vi "channel cluster to array.vi"(11 "input cluster":T1 {"Vfile (V)" format="%.1f V"; "Vswmax (V)" format="%#_g V"; "Iset (A)" format="%.2pA"; "Imon (A)" format="%.2pA"; "Vset (V)" format="%#_g V"; "Vmon (V)" format="%.1f V"}) -> (3 "Array":string[](array[string]))   [LabVIEW 2018]
uses:
  channel_cluster.ctl
  bool to string small.vi
  dbl to fr string small.vi
  i32 to dec string small.vi
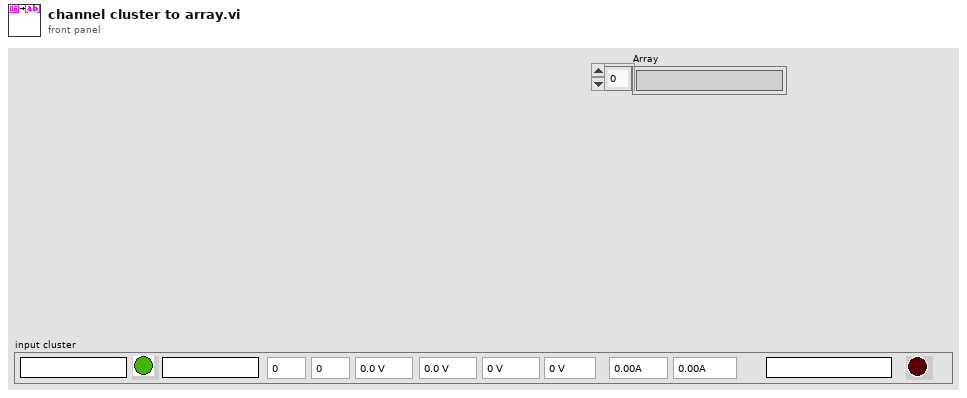
[diagram p1: front panel]
types:
  T1 = typedef "channel_cluster.ctl" = cluster{"Channel Name":string, "Crate":i32, "Card Type":string, "Card":i32, "Channel":i32, "Status Icon":picture, "Vmon (V)":dbl, "Vset (V)":dbl, "Imon (A)":dbl, "Iset (A)":dbl, "Timestamp":string, "ON/OFF":bool, "Status":string, "Vswmax (V)":dbl, "Flag":bool, "Vfile (V)":dbl, "Error Logged":bool[], "enable_file":bool}
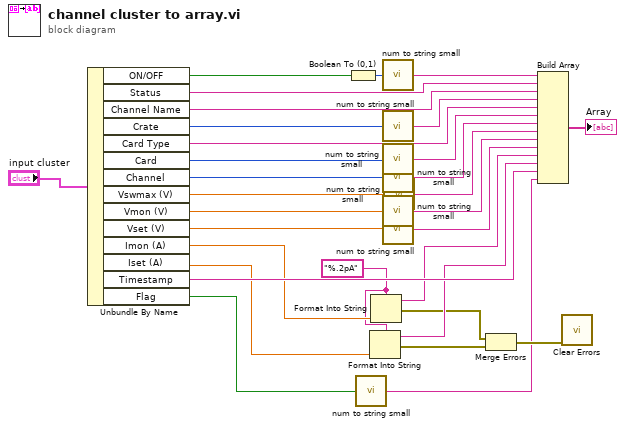
[diagram p0: block diagram]
diagram:
  w6 = "%.2pA" ("format string")
  n1 = Unbundle By Name("input cluster") -> ("ON/OFF"=w14:bool, "Status"=w17:string, "Channel Name"=w20:string, "Crate"=w21:i32, "Card Type"=w22:string, "Card"=w23:i32, "Channel"=w24:i32, "Vswmax (V)"=w12:dbl, "Vmon (V)"=w18:dbl, "Vset (V)"=w19:dbl, "Imon (A)"=w7:dbl, "Iset (A)"=w8:dbl, "Timestamp"=w29:string, "Flag"=w2:bool)
  n2 = Boolean To (0,1)(Boolean=w14) -> (0, 1=w15:i16)
  n3 = call-poly "num to string small.vi"("number"=w2) -> ("String"=w1:string)  [unwired: 14 in]
  n4 = Format Into String(format string=w6, w8) -> (resulting string=w9:string, error out=w4:errorcluster)  [unwired: 2 in]
  n5 = Format Into String(format string=w6, w7) -> (resulting string=w10:string, error out=w5:errorcluster)  [unwired: 2 in]
  n6 = call-poly "num to string small.vi"("number"=w15) -> ("String"=w16:string)  [unwired: 14 in]
  n7 = call-poly "num to string small.vi"("number"=w21) -> ("String"=w13:string)  [unwired: 14 in]
  n8 = call-poly "num to string small.vi"("number"=w23) -> ("String"=w25:string)  [unwired: 14 in]
  n9 = call-poly "num to string small.vi"("number"=w24) -> ("String"=w26:string)  [unwired: 14 in]
  n10 = call-poly "num to string small.vi"("number"=w18) -> ("String"=w27:string)  [unwired: 14 in]
  n11 = call-poly "num to string small.vi"("number"=w19) -> ("String"=w28:string)  [unwired: 14 in]
  n12 = call-poly "num to string small.vi"("number"=w12) -> ("String"=w11:string)  [unwired: 14 in]
  n13 = Merge Errors(w5, w4) -> (w3:errorcluster)
  n14 = Build Array(w16, w17, w20, w13, w22, w25, w26, w11, w27, w28, w10, w9, w29, w1) -> (→"Array":string[])
  n15 = call <vilib>:"Clear Errors.vi"("error in (no error)"=w3) -> ()  [unwired: 5 in, 2 out]
